vi "AD（V3.2）.vi"(8 "N-length":dbl, 9 "M-length":dbl, 10 "hDevice":i32) -> (0 "幅频谱":dbl[](graph), 1 "时域谱":dbl[](graph), 3 "hDevice out":i32)   [LabVIEW 2016]
uses:
  ACTS1001_32.dll
panel:
  out "CH0 Data (mV)":sgl[](graph)
  out "使能通道总数":i32
  out "CH2 Data (mV)":sgl[](graph)
  out "CH3 Data (mV)":sgl[](graph)
  out "CH1 Data (mV)":sgl[](graph)
  in  "停止 2":bool
  in  "量程选择 7":i32(ring) items=["±5000mV"=0, "±1000mV"=2]
  in  "量程选择 6":i32(ring) items=["±5000mV"=0, "±1000mV"=2]
  in  "量程选择 5":i32(ring) items=["±5000mV"=0, "±1000mV"=2]
  in  "量程选择 4":i32(ring) items=["±5000mV"=0, "±1000mV"=2]
  in  "停止":bool
  in  "量程选择 3":i32(ring) items=["±5000mV"=0, "±1000mV"=2]
  in  "量程选择 2":i32(ring) items=["±5000mV"=0, "±1000mV"=2]
  in  "量程选择 1":i32(ring) items=["±5000mV"=0, "±1000mV"=2]
  in  "量程选择 0":i32(ring) items=["±5000mV"=0, "±1000mV"=2]
  out "要读取和处理的AD数据长度":u32
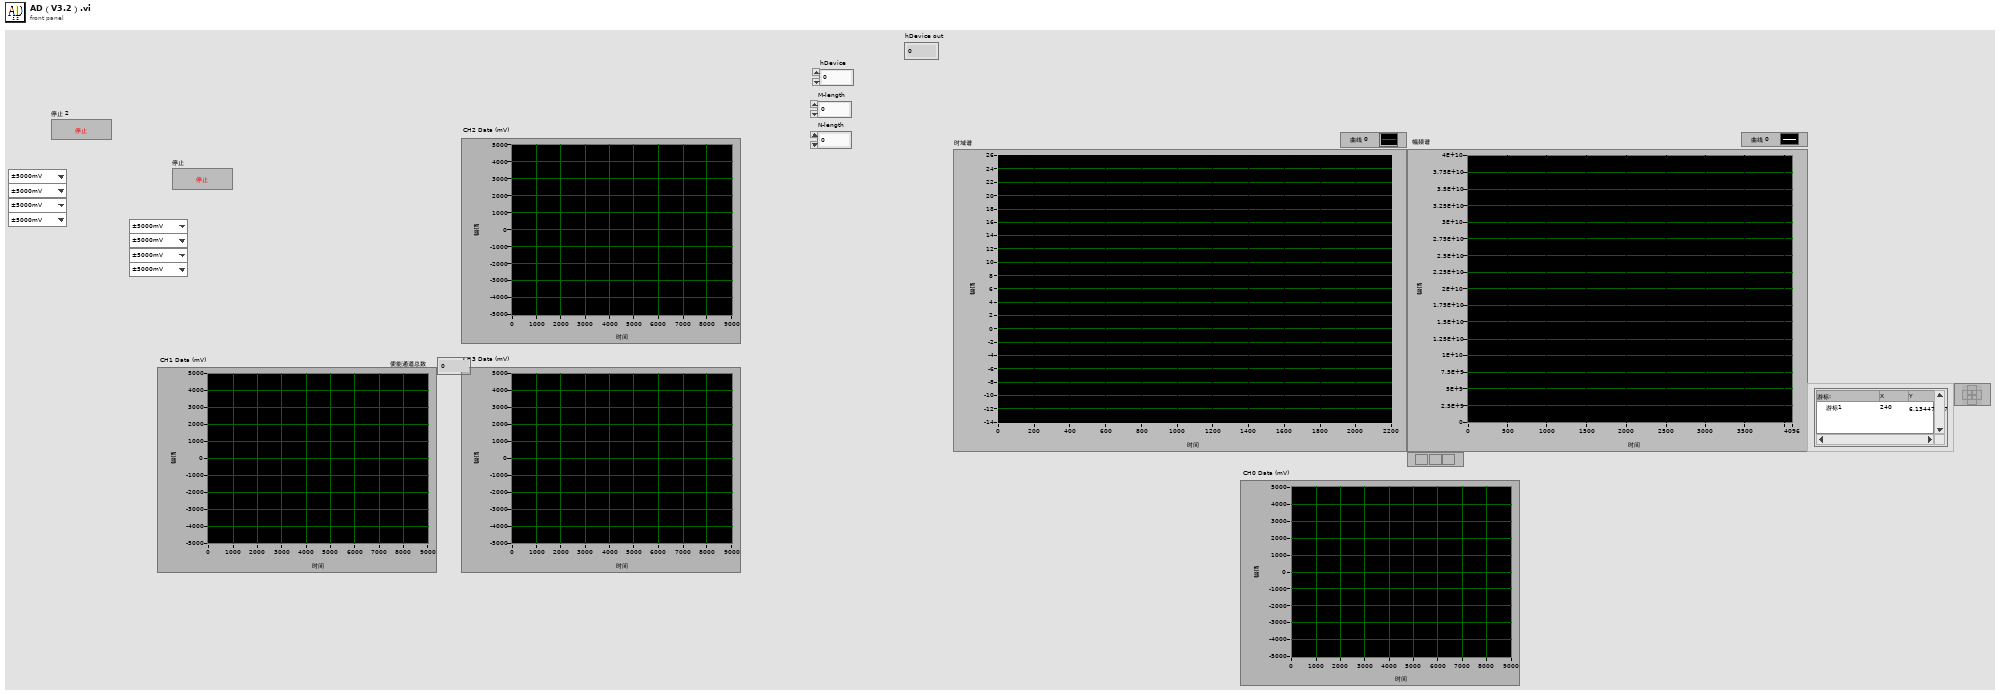
[diagram p1: front panel]
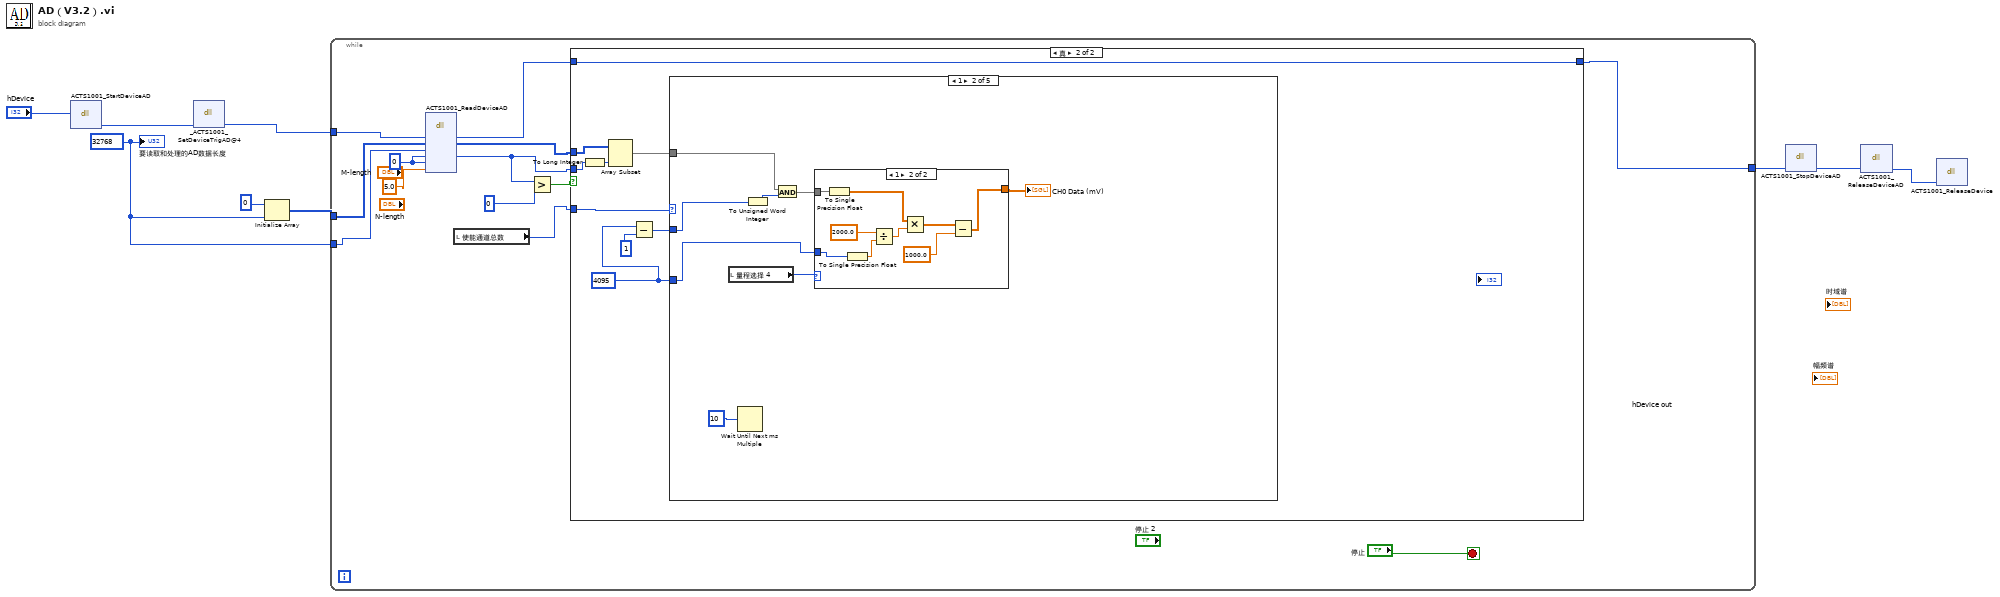
[diagram p0: block diagram]
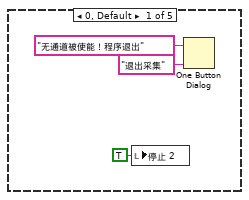
[diagram p3: hidden frame]
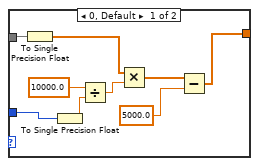
[diagram p4: hidden frame]
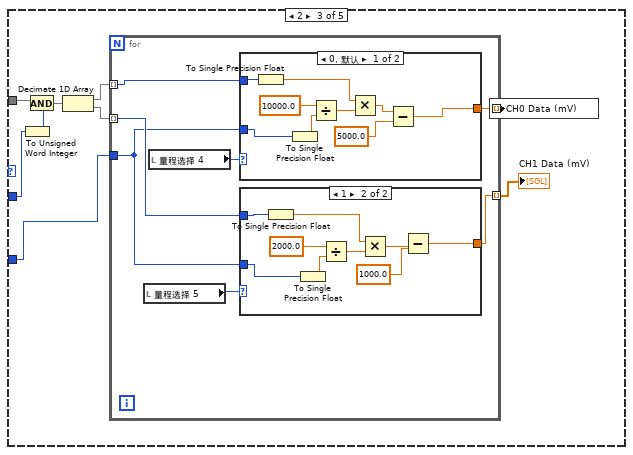
[diagram p5: hidden frame]
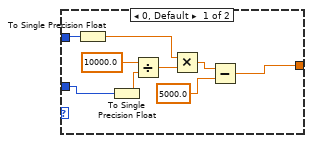
[diagram p6: hidden frame]
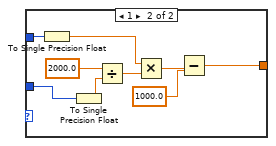
[diagram p7: hidden frame]
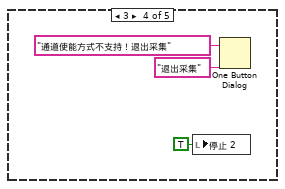
[diagram p8: hidden frame]
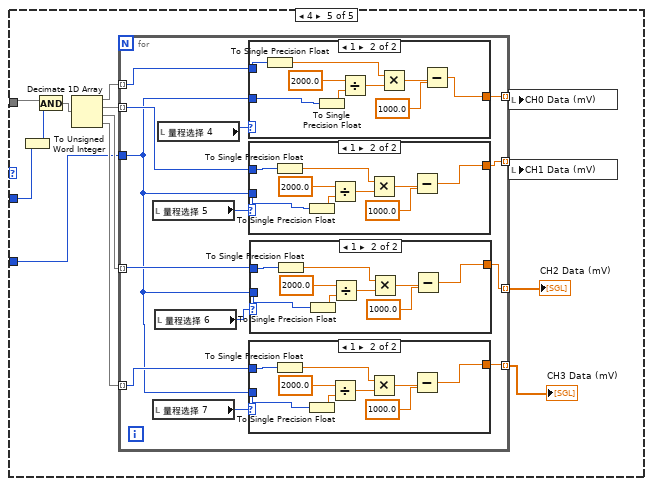
[diagram p9: hidden frame]
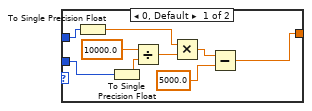
[diagram p10: hidden frame]
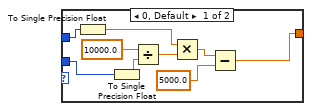
[diagram p11: hidden frame]
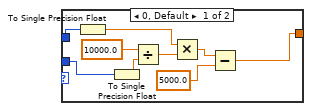
[diagram p12: hidden frame]
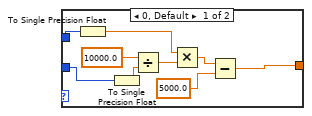
[diagram p13: hidden frame]
diagram:
  w4 = u32 32768 ("采样编码数量 2")
  n1 = dll-call lib="ACTS1001_32.dll" fn="ACTS1001_StartDeviceAD"("hDevice"="hDevice") -> ("hDevice"=w8:i32)  [unwired: 4 in, 2 out]
  n2 = dll-call lib="ACTS1001_32.dll" fn="_ACTS1001_SetDeviceTrigAD@4" label="ACTS1001_SetDeviceTrigAD"("hDevice"=w8) -> ("hDevice"=w6:i32)  [unwired: 4 in, 2 out]
  n3 = Initialize Array(u16 0, w4) -> (w5:u16[])
  n4 = while {
    tunnel: w6 -> [w23]
    tunnel: w5 -> [w22]
    tunnel: w4 -> [w21]
    tunnel: [w11] -> w1
    stop <- "停止" stop-if-true
    w20 = u16 0
    n5 = dll-call lib="ACTS1001_32.dll" fn="ACTS1001_ReadDeviceAD"("hDevice"=w23, "pADBuffer"=w22, "nReadSizeWords"=w21, "nRetSizeWords"=w20, "pAvailSampsPoints"=w20, "fTimeout"=5.0) -> ("hDevice"=w18:i32, "pADBuffer"=w17:u16[], "nRetSizeWords"=w14:u32)  [unwired: 7 in, 2 out]
    n6 = local read "使能通道总数"() -> (w16:i32)
    n7 = Greater?(x=w14, y=u16 0) -> (0:w15:bool)
    n8 = case shown="真" w15 {
      tunnel: w18 -> [w24 w33]
      tunnel: [w24 w33] -> w11
      tunnel: w17 -> [_ w30]
      tunnel: w14 -> [_ w28]
      tunnel: w16 -> [_ w32]
      frame False {
      }
      frame True {
        w25 = u16 4095
        n9 = To Long Integer(number=w28) -> (32bit integer=w31:i32)
        n10 = Array Subset(array=w30, length=w31) -> (w29:u16[])  [unwired: 1 in]
        n11 = Subtract(x=w25, y=1) -> (x-y=w26:i32)
        n12 = case shown="1" w32 {
          tunnel: w29 -> [_ w40 w67 _ w125]
          tunnel: w26 -> [_ w38 w62 _ w118]
          tunnel: w25 -> [_ w39 w63 _ w117]
          frame 0, Default {
            n13 = local write "停止 2"(TRUE ("停止")) -> ()
            n14 = One Button Dialog(message="无通道被使能！程序退出" ("消息"), button name ("OK")="退出采集" ("按钮名称（“确定”）")) -> ()  [unwired: 1 out]
          }
          frame 1 {
            n15 = local read "量程选择 4"() -> (w41:i32)
            n16 = To Unsigned Word Integer(number=w38) -> (unsigned 16bit integer=w42:u16)
            n17 = And(x=w40, y=w42) -> (x .and. y?=w43:u16[])
            n18 = case shown="1" w41 {
              tunnel: w43 -> [w52 w61]
              tunnel: [w47 w56] -> w37
              tunnel: w39 -> [w44 w53]
              frame 0, Default {
                n19 = To Single Precision Float(number=w52) -> (single precision float=w50:sgl[])
                n20 = To Single Precision Float(number=w44) -> (single precision float=w45:sgl)
                n21 = Divide(x=sgl 10000.0, y=w45) -> (x/y=w51:sgl)
                n22 = Multiply(x=w50, y=w51) -> (x*y=w49:sgl[])
                n23 = Subtract(x=w49, y=sgl 5000.0) -> (x-y=w47:sgl[])
              }
              frame 1 {
                n24 = To Single Precision Float(number=w61) -> (single precision float=w59:sgl[])
                n25 = To Single Precision Float(number=w53) -> (single precision float=w54:sgl)
                n26 = Divide(x=sgl 2000.0, y=w54) -> (x/y=w60:sgl)
                n27 = Multiply(x=w59, y=w60) -> (x*y=w58:sgl[])
                n28 = Subtract(x=w58, y=sgl 1000.0) -> (x-y=w56:sgl[])
              }
            }
            "CH0 Data (mV)" <- w37
          }
          frame 2 {
            n29 = To Unsigned Word Integer(number=w62) -> (unsigned 16bit integer=w68:u16)
            n30 = And(x=w67, y=w68) -> (x .and. y?=w66:u16[])
            n31 = Decimate 1D Array(w66) -> (w70:u16[], w69:u16[])
            n32 = for {
              tunnel: w70 -> [w76] mode=indexing
              tunnel: w69 -> [w74] mode=indexing
              tunnel: w63 -> [w73]
              tunnel: [w72] -> w65 mode=indexing
              tunnel: [w71] -> w64 mode=indexing
              n33 = local read "量程选择 5"() -> (w75:i32)
              n34 = local read "量程选择 4"() -> (w77:i32)
              n35 = case shown="0, 默认" w77 {
                tunnel: w76 -> [w104 w113]
                tunnel: [w99 w108] -> w72
                tunnel: w73 -> [w96 w105]
                frame 0, Default {
                  n36 = To Single Precision Float(number=w104) -> (single precision float=w102:sgl)
                  n37 = To Single Precision Float(number=w96) -> (single precision float=w97:sgl)
                  n38 = Divide(x=sgl 10000.0, y=w97) -> (x/y=w103:sgl)
                  n39 = Multiply(x=w102, y=w103) -> (x*y=w101:sgl)
                  n40 = Subtract(x=w101, y=sgl 5000.0) -> (x-y=w99:sgl)
                }
                frame 1 {
                  n41 = To Single Precision Float(number=w113) -> (single precision float=w111:sgl)
                  n42 = To Single Precision Float(number=w105) -> (single precision float=w106:sgl)
                  n43 = Divide(x=sgl 2000.0, y=w106) -> (x/y=w112:sgl)
                  n44 = Multiply(x=w111, y=w112) -> (x*y=w110:sgl)
                  n45 = Subtract(x=w110, y=sgl 1000.0) -> (x-y=w108:sgl)
                }
              }
              n46 = case shown="1" w75 {
                tunnel: w74 -> [w86 w95]
                tunnel: [w81 w90] -> w71
                tunnel: w73 -> [w78 w87]
                frame 0, Default {
                  n47 = To Single Precision Float(number=w86) -> (single precision float=w84:sgl)
                  n48 = To Single Precision Float(number=w78) -> (single precision float=w79:sgl)
                  n49 = Divide(x=sgl 10000.0, y=w79) -> (x/y=w85:sgl)
                  n50 = Multiply(x=w84, y=w85) -> (x*y=w83:sgl)
                  n51 = Subtract(x=w83, y=sgl 5000.0) -> (x-y=w81:sgl)
                }
                frame 1 {
                  n52 = To Single Precision Float(number=w95) -> (single precision float=w93:sgl)
                  n53 = To Single Precision Float(number=w87) -> (single precision float=w88:sgl)
                  n54 = Divide(x=sgl 2000.0, y=w88) -> (x/y=w94:sgl)
                  n55 = Multiply(x=w93, y=w94) -> (x*y=w92:sgl)
                  n56 = Subtract(x=w92, y=sgl 1000.0) -> (x-y=w90:sgl)
                }
              }
            }
            "CH1 Data (mV)" <- w64
            n57 = local write "CH0 Data (mV)"(w65) -> ()
          }
          frame 3 {
            n58 = local write "停止 2"(TRUE ("停止")) -> ()
            n59 = One Button Dialog(message="通道使能方式不支持！退出采集" ("消息"), button name ("OK")="退出采集" ("按钮名称（“确定”）")) -> ()  [unwired: 1 out]
          }
          frame 4 {
            n60 = To Unsigned Word Integer(number=w118) -> (unsigned 16bit integer=w127:u16)
            n61 = And(x=w125, y=w127) -> (x .and. y?=w126:u16[])
            n62 = Decimate 1D Array(w126) -> (w129:u16[], w128:u16[], w124:u16[], w123:u16[])
            n63 = for {
              tunnel: w129 -> [w141] mode=indexing
              tunnel: w128 -> [w139] mode=indexing
              tunnel: w117 -> [w130]
              tunnel: [w138] -> w120 mode=indexing
              tunnel: [w137] -> w119 mode=indexing
              tunnel: w124 -> [w136] mode=indexing
              tunnel: w123 -> [w135] mode=indexing
              tunnel: [w134] -> w122 mode=indexing
              tunnel: [w133] -> w121 mode=indexing
              n64 = local read "量程选择 5"() -> (w140:i32)
              n65 = local read "量程选择 7"() -> (w131:i32)
              n66 = local read "量程选择 6"() -> (w132:i32)
              n67 = local read "量程选择 4"() -> (w142:i32)
              n68 = case shown="1" w142 {
                tunnel: w141 -> [w205 w214]
                tunnel: [w200 w209] -> w138
                tunnel: w130 -> [w197 w206]
                frame 0, Default {
                  n69 = To Single Precision Float(number=w205) -> (single precision float=w203:sgl)
                  n70 = To Single Precision Float(number=w197) -> (single precision float=w198:sgl)
                  n71 = Divide(x=sgl 10000.0, y=w198) -> (x/y=w204:sgl)
                  n72 = Multiply(x=w203, y=w204) -> (x*y=w202:sgl)
                  n73 = Subtract(x=w202, y=sgl 5000.0) -> (x-y=w200:sgl)
                }
                frame 1 {
                  n74 = To Single Precision Float(number=w214) -> (single precision float=w212:sgl)
                  n75 = To Single Precision Float(number=w206) -> (single precision float=w207:sgl)
                  n76 = Divide(x=sgl 2000.0, y=w207) -> (x/y=w213:sgl)
                  n77 = Multiply(x=w212, y=w213) -> (x*y=w211:sgl)
                  n78 = Subtract(x=w211, y=sgl 1000.0) -> (x-y=w209:sgl)
                }
              }
              n79 = case shown="1" w140 {
                tunnel: w139 -> [w187 w196]
                tunnel: [w182 w191] -> w137
                tunnel: w130 -> [w179 w188]
                frame 0, Default {
                  n80 = To Single Precision Float(number=w187) -> (single precision float=w185:sgl)
                  n81 = To Single Precision Float(number=w179) -> (single precision float=w180:sgl)
                  n82 = Divide(x=sgl 10000.0, y=w180) -> (x/y=w186:sgl)
                  n83 = Multiply(x=w185, y=w186) -> (x*y=w184:sgl)
                  n84 = Subtract(x=w184, y=sgl 5000.0) -> (x-y=w182:sgl)
                }
                frame 1 {
                  n85 = To Single Precision Float(number=w196) -> (single precision float=w194:sgl)
                  n86 = To Single Precision Float(number=w188) -> (single precision float=w189:sgl)
                  n87 = Divide(x=sgl 2000.0, y=w189) -> (x/y=w195:sgl)
                  n88 = Multiply(x=w194, y=w195) -> (x*y=w193:sgl)
                  n89 = Subtract(x=w193, y=sgl 1000.0) -> (x-y=w191:sgl)
                }
              }
              n90 = case shown="1" w131 {
                tunnel: w135 -> [w151 w160]
                tunnel: [w146 w155] -> w134
                tunnel: w130 -> [w143 w152]
                frame 0, Default {
                  n91 = To Single Precision Float(number=w151) -> (single precision float=w149:sgl)
                  n92 = To Single Precision Float(number=w143) -> (single precision float=w144:sgl)
                  n93 = Divide(x=sgl 10000.0, y=w144) -> (x/y=w150:sgl)
                  n94 = Multiply(x=w149, y=w150) -> (x*y=w148:sgl)
                  n95 = Subtract(x=w148, y=sgl 5000.0) -> (x-y=w146:sgl)
                }
                frame 1 {
                  n96 = To Single Precision Float(number=w160) -> (single precision float=w158:sgl)
                  n97 = To Single Precision Float(number=w152) -> (single precision float=w153:sgl)
                  n98 = Divide(x=sgl 2000.0, y=w153) -> (x/y=w159:sgl)
                  n99 = Multiply(x=w158, y=w159) -> (x*y=w157:sgl)
                  n100 = Subtract(x=w157, y=sgl 1000.0) -> (x-y=w155:sgl)
                }
              }
              n101 = case shown="1" w132 {
                tunnel: w136 -> [w162 w178]
                tunnel: [w165 w173] -> w133
                tunnel: w130 -> [w161 w170]
                frame 0, Default {
                  n102 = To Single Precision Float(number=w162) -> (single precision float=w168:sgl)
                  n103 = To Single Precision Float(number=w161) -> (single precision float=w163:sgl)
                  n104 = Divide(x=sgl 10000.0, y=w163) -> (x/y=w169:sgl)
                  n105 = Multiply(x=w168, y=w169) -> (x*y=w167:sgl)
                  n106 = Subtract(x=w167, y=sgl 5000.0) -> (x-y=w165:sgl)
                }
                frame 1 {
                  n107 = To Single Precision Float(number=w178) -> (single precision float=w176:sgl)
                  n108 = To Single Precision Float(number=w170) -> (single precision float=w171:sgl)
                  n109 = Divide(x=sgl 2000.0, y=w171) -> (x/y=w177:sgl)
                  n110 = Multiply(x=w176, y=w177) -> (x*y=w175:sgl)
                  n111 = Subtract(x=w175, y=sgl 1000.0) -> (x-y=w173:sgl)
                }
              }
            }
            "CH2 Data (mV)" <- w121
            "CH3 Data (mV)" <- w122
            n112 = local write "CH0 Data (mV)"(w120) -> ()
            n113 = local write "CH1 Data (mV)"(w119) -> ()
          }
        }
      }
    }
  }
  n114 = Wait Until Next ms Multiple(millisecond multiple=u32 10) -> ()  [unwired: 1 out]
  n115 = dll-call lib="ACTS1001_32.dll" fn="ACTS1001_StopDeviceAD" label="StopDeviceAD"("hDevice"=w1) -> ("hDevice"=w3:i32)  [unwired: 4 in, 2 out]
  n116 = dll-call lib="ACTS1001_32.dll" fn="ACTS1001_ReleaseDeviceAD" label="ReleaseDeviceAD"("hDevice"=w3) -> ("hDevice"=w2:i32)  [unwired: 4 in, 2 out]
  n117 = dll-call lib="ACTS1001_32.dll" fn="ACTS1001_ReleaseDevice" label="ReleaseDevice"("hDevice"=w2) -> ()  [unwired: 5 in, 2 out]
  "要读取和处理的AD数据长度" <- w4
